vi "L1OC_Phase_computatio_NIRS.vi"() -> (6 "Массив индексов фазы кода":i32[](array[numeric]))   [LabVIEW 2020]
uses:
  <vilib>/Analysis/2dsp.llb/Complex FFT.vi
  <vilib>/measure/maspectr.llb/FFT Power Spectrum and PSD for 1 Chan (CDB).vi
  <vilib>/Analysis/NI_AALPro.lvlib
  <vilib>/measure/NI_MAPro.lvlib
  <vilib>/Analysis/NI_AALBase.lvlib
panel:
  in  "Длительность сигнала":i32=50
  in  "Время моделирование 1023 символов":dbl=0.008
  in  "Длина ПСП":dbl=1023.0
  in  "file path (use dialog)":path=path "C:/Users/ira_1/OneDrive/Рабочий стол/samples.bin"
  in  "qc/N0":dbl=50.0
  out "Waveform Graph 3":cluster{"f0":dbl, "df":dbl, "magnitude":dbl[]}(graph)
  out "Waveform Graph 2":waveform(dbl)(graph)
  in  "stop":bool
  in  "Частота\n дикретизации, Гц":dbl=5000000.0
  in  "Доплер\nнесущей, Гц":dbl=1000.0
  in  "Несущая\nчастота, Гц":dbl=1575450000.0
  in  "Задержка\nкода, симв":dbl=1.0
  out "Waveform Graph":dbl[](graph)
  out "Array":cdb[](array[numeric])
  out "доплер нес":dbl
  out "доплер код":dbl
  out "index of element":i32
  # "Блок вычисления фазы кода для составного сигнала КА"
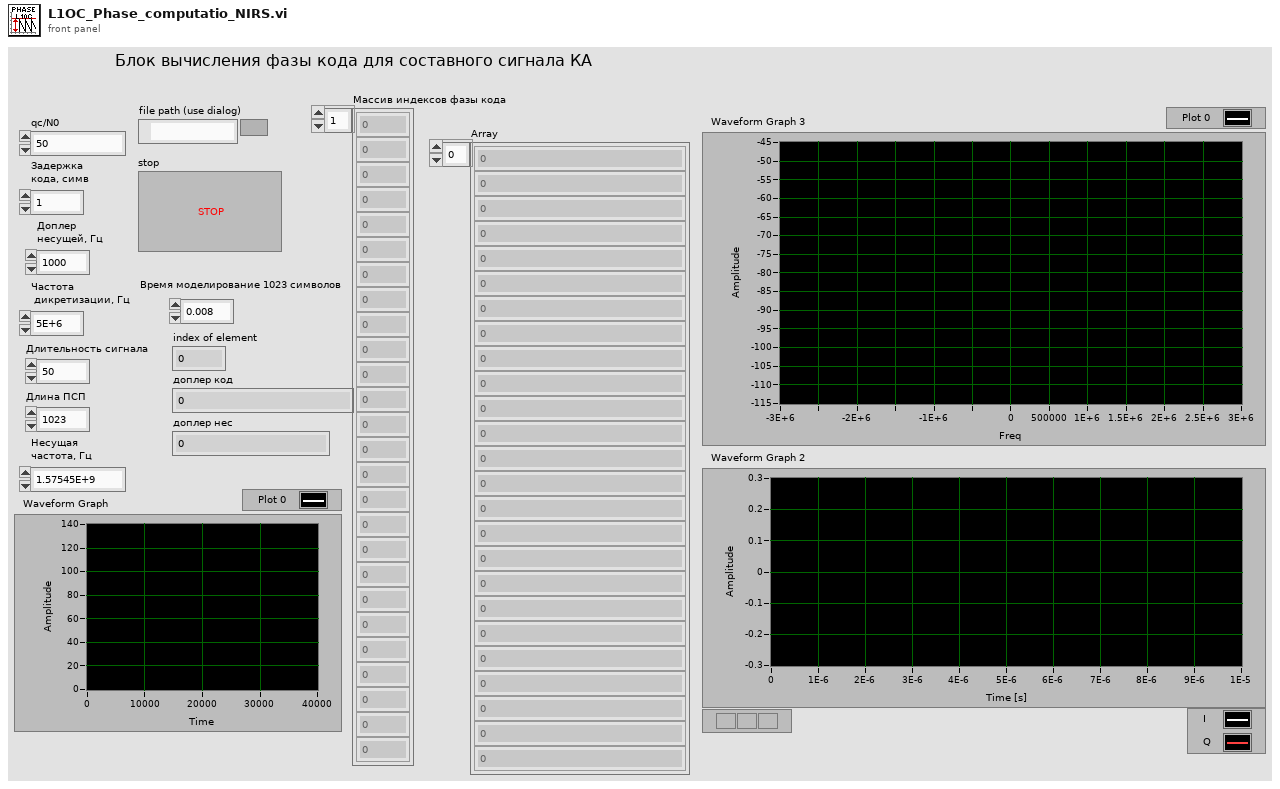
[diagram p1: front panel]
types:
  T1 = enum16{"open", "replace", "create", "open or create", "replace or create", "replace or create with confirmation"}
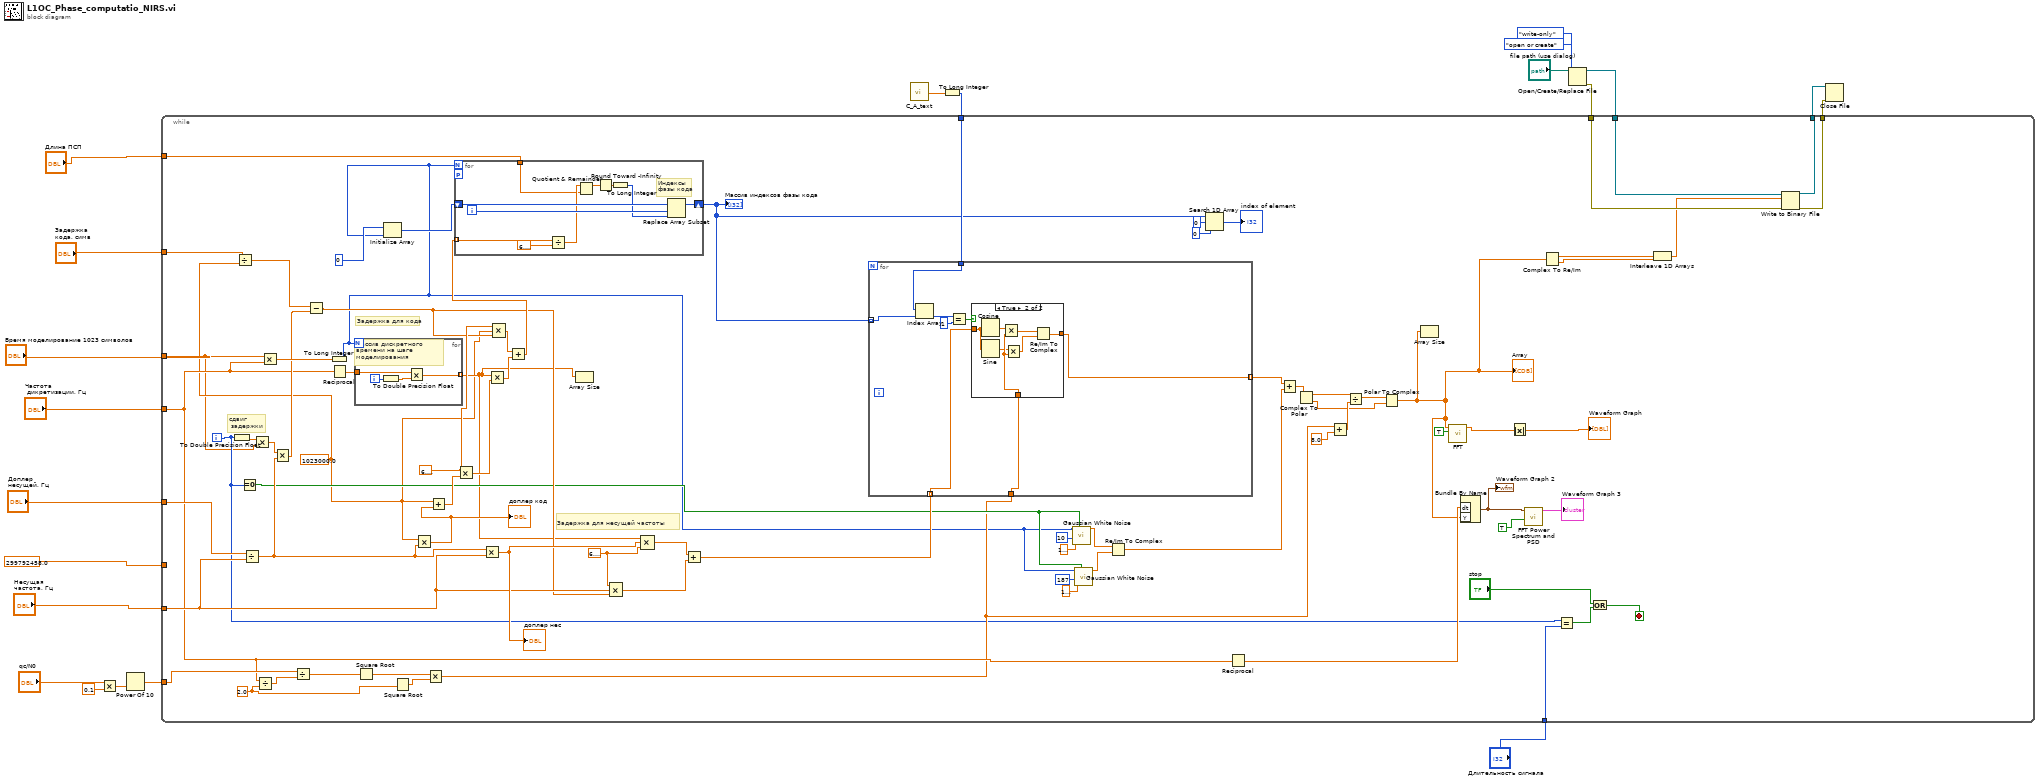
[diagram p0: block diagram]
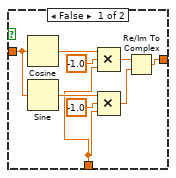
[diagram p2: hidden frame]
diagram:
  n1 = Multiply(x="qc/N0", y=0.1) -> (x*y=w14:dbl)
  n2 = Power Of 10(x=w14) -> (10^x=w13:dbl)
  n3 = call "C_A_text.vi"() -> ("array"=w5:dbl[])  [unwired: 2 in]
  n4 = To Long Integer(number=w5) -> (32bit integer=w4:i32[])
  n5 = Open/Create/Replace File(file path (use dialog)="file path (use dialog)", operation (0:open)=T1."open or create", access (0:read/write)=enum16{"read/write", "read-only", "write-only"}."write-only") -> (refnum out=w11:refnum<file>, error out=w8:errorcluster)  [unwired: 3 in, 1 out]
  n6 = while {
    tunnel: "Время моделирование 1023 символов" -> [w24]
    tunnel: w4 -> [w89]
    tunnel: "Задержка\nкода, симв" -> [w76]
    tunnel: "Доплер\nнесущей, Гц" -> [w73]
    tunnel: 299792458.0 ("y") -> [_]
    tunnel: "Несущая\nчастота, Гц" -> [w68]
    tunnel: "Частота\n дикретизации, Гц" -> [w53]
    tunnel: w13 -> [w62]
    tunnel: w11 -> [w37]
    tunnel: w8 -> [w36]
    tunnel: [w35] -> w7
    tunnel: [w34] -> w6
    tunnel: "Длина ПСП" -> [w23]
    tunnel: "Длительность сигнала" -> [w22]
    i -> [w30]
    stop <- w38 stop-if-true
    w29 = 2.0
    w78 = 6.283185307179586
    w25 = 1023000.0 ("value")
    w97 = 6.283185307179586
    # "сдвиг\n задержки"
    # "Задержка для кода"
    # "Задержка для несущей частоты"
    n7 = To Double Precision Float(number=w30) -> (double precision float=w75:dbl)
    n8 = Divide(x=w76, y=w25) -> (x/y=w63:dbl)
    n9 = Equal To 0?(x=w30) -> (x = 0?=w56:bool)
    n10 = Divide(x=w73, y=w68) -> (x/y=w72:dbl)
    n11 = Multiply(x=w75, y=w24) -> (x*y=w74:dbl)
    n12 = Divide(x=w53, y=w29) -> (x/y=w52:dbl)
    n13 = Multiply(x=w24, y=w53) -> (x*y=w99:dbl)
    n14 = Multiply(x=w74, y=w72) -> (x*y=w64:dbl)
    n15 = Divide(x=w62, y=w52) -> (x/y=w61:dbl)
    n16 = Subtract(x=w63, y=w64) -> (x-y=w65:dbl)
    n17 = To Long Integer(number=w99) -> (32bit integer=w26:i32)
    n18 = Reciprocal(x=w53) -> (1/x=w98:dbl)
    n19 = for {
      N: w26 -> [_]
      tunnel: w98 -> [w125]
      tunnel: [w124] -> w27 mode=indexing
      i -> [w127]
      # "массив дискретного \nвремени на шаге \nмоделирования"
      n20 = To Double Precision Float(number=w127) -> (double precision float=w126:dbl)
      n21 = Multiply(x=w125, y=w126) -> (x*y=w124:dbl)
    }
    n22 = Square Root(x=w61) -> (sqrt(x)=w60:dbl)
    n23 = Initialize Array(0, w26) -> (w90:i32[])
    n24 = Square Root(x=w29) -> (sqrt(x)=w59:dbl)
    n25 = Multiply(x=w25, y=w72) -> (x*y=w66:dbl)
    "доплер код" <- w66
    n26 = Multiply(x=w60, y=w59) -> (x*y=w47:dbl)
    n27 = Add(x=w25, y=w66) -> (x+y=w96:dbl)
    n28 = Multiply(x=w97, y=w96) -> (x*y=w95:dbl)
    n29 = Multiply(x=w72, y=w68) -> (x*y=w77:dbl)
    "доплер нес" <- w77
    n30 = Multiply(x=w27, y=w95) -> (x*y=w94:dbl[])
    n31 = Compound Arithmetic op=MULTIPLY(w97, w25, w65) -> (w93:dbl)
    n32 = Add(x=w93, y=w94) -> (x+y=w92:dbl[])
    n33 = for {
      N: w26 -> [_]
      shift-right: [w135] -> w88
      shift-left: w90 -> [w134]
      workers-P: _ -> [_]
      tunnel: w92 -> [w131] mode=indexing
      tunnel: w23 -> [w128]
      i -> [w133]
      # "Индексы\nфазы кода"
      n34 = Divide(x=w131, y=6.283185307179586) -> (x/y=w129:dbl)
      n35 = Quotient & Remainder(x=w129, y=w128) -> (x-y*floor(x/y)=w136:dbl)  [unwired: 1 out]
      n36 = Round Toward -Infinity(1:w136) -> (0:w137:dbl)
      n37 = To Long Integer(number=w137) -> (32bit integer=w132:i32)
      n38 = Replace Array Subset(array=w134, new element=w132, index=w133) -> (w135:i32[])
    }
    "Массив индексов фазы кода" <- w88
    n39 = Array Size(array=w27) -> ()  [unwired: 1 out]
    n40 = Compound Arithmetic op=MULTIPLY(w78, w68, w65) -> (w84:dbl)
    n41 = Compound Arithmetic op=MULTIPLY(w27, w77, w78) -> (w79:dbl[])
    n42 = Add(x=w79, y=w84) -> (x+y=w83:dbl[])
    n43 = for {
      tunnel: w89 -> [w107]
      tunnel: w88 -> [w106] mode=indexing
      tunnel: w83 -> [w102] mode=indexing
      tunnel: [w101] -> w48 mode=indexing
      tunnel: w47 -> [w100]
      n44 = Index Array(array=w107, index=w106) -> (element=w105:i32)
      n45 = Equal?(x=w105, y=1) -> (x = y?=w103:bool)
      n46 = case shown="True" w103 {
        tunnel: w102 -> [w116 w123]
        tunnel: [w115 w122] -> w101
        tunnel: w100 -> [w110 w119]
        frame False {
          n47 = Cosine(x=w116) -> (cos(x)=w113:dbl)
          n48 = Sine(x=w116) -> (sin(x)=w111:dbl)
          n49 = Compound Arithmetic op=MULTIPLY(w113, -1.0 ("y"), w110) -> (w108:dbl)
          n50 = Compound Arithmetic op=MULTIPLY(w111, -1.0 ("y"), w110) -> (w109:dbl)
          n51 = Re/Im To Complex(1:w109, 2:w108) -> (0:w115:cdb)
        }
        frame True {
          n52 = Cosine(x=w123) -> (cos(x)=w121:dbl)
          n53 = Sine(x=w123) -> (sin(x)=w118:dbl)
          n54 = Multiply(x=w121, y=w119) -> (x*y=w120:dbl)
          n55 = Multiply(x=w118, y=w119) -> (x*y=w117:dbl)
          n56 = Re/Im To Complex(1:w117, 2:w120) -> (0:w122:cdb)
        }
      }
    }
    n57 = call <vilib>:"Gaussian White Noise.vi"("initialize?"=w56, "seed"=10, "standard deviation"=1.0000000000000002, "samples"=w26) -> ("Gaussian noise pattern"=w51:dbl[])  [unwired: 6 in, 1 out]
    n58 = call <vilib>:"Gaussian White Noise.vi"("initialize?"=w56, "seed"=187, "standard deviation"=1.0000000000000002, "samples"=w26) -> ("Gaussian noise pattern"=w50:dbl[])  [unwired: 6 in, 1 out]
    n59 = Re/Im To Complex(1:w50, 2:w51) -> (0:w49:cdb[])
    n60 = Search 1D Array(1D array=w88, element=0, start index (0)=0) -> (index of element=→"index of element":i32)
    n61 = Reciprocal(x=w53) -> (1/x=w67:dbl)
    n62 = Add(x=w48, y=w49) -> (x+y=w45:cdb[])
    n63 = Complex To Polar(r * e^(i*theta)=w45) -> (r=w44:dbl[], theta=w41:dbl[])
    n64 = Add(x=w47, y=8.0) -> (x+y=w43:dbl)
    n65 = Divide(x=w44, y=w43) -> (x/y=w42:dbl[])
    n66 = Polar To Complex(1:w41, 2:w42) -> (0:w28:cdb[])
    "Array" <- w28
    n67 = Array Size(array=w28) -> ()  [unwired: 1 out]
    n68 = call-poly <vilib>:"FFT.vi"("shift?"=TRUE, "X"=w28) -> ("FFT {X}"=w81:cdb[])  [unwired: 8 in, 1 out]
    n69 = Bundle By Name("dt"=w67, "Y"=w28) -> (w69:waveform(cdb))  [unwired: 1 in]
    "Waveform Graph 2" <- w69
    n70 = Absolute Value(x=w81) -> (abs(x)=→"Waveform Graph":dbl[])
    n71 = call-poly <vilib>:"FFT Power Spectrum and PSD.vi"("dB On (F)"=TRUE, "time signal"=w69) -> ("Power Spectrum / PSD"=→"Waveform Graph 3":cluster{"f0":dbl, "df":dbl, "magnitude":dbl[]})  [unwired: 6 in, 3 out]
    n72 = Complex To Re/Im(x + iy=w28) -> (x=w33:dbl[], y=w32:dbl[])
    n73 = Equal?(x=w30, y=w22) -> (x = y?=w39:bool)
    n74 = Or(x="stop", y=w39) -> (x .or. y?=w38:bool)
    n75 = Interleave 1D Arrays(w33, w32) -> (w31:dbl[])
    n76 = Write to Binary File(file (use dialog)=w37, data=w31, error in=w36) -> (refnum out=w35:refnum<file>, error out=w34:errorcluster)  [unwired: 3 in, 1 out]
  }
  n77 = Close File(refnum=w7, error in=w6) -> ()  [unwired: 2 out]
